vi "F5xxx Set Level.vi"(8 "error in (no error)":errorcluster, 9 "level [V/A]":dbl format="%^.3e", 10 "f [Hz]":dbl min=0.0 max=1200000.0 format="%^.3e", 11 "session in":T1) -> (0 "error out":errorcluster, 3 "session out":T1)   [LabVIEW 2020]
doc: "Set Fluke 5xxx voltage or current level."
uses:
  F5xxx_session.ctl
  F5xxx_output_mode.ctl
  Fluke 5XXX Series Multicalibrators.lvlib
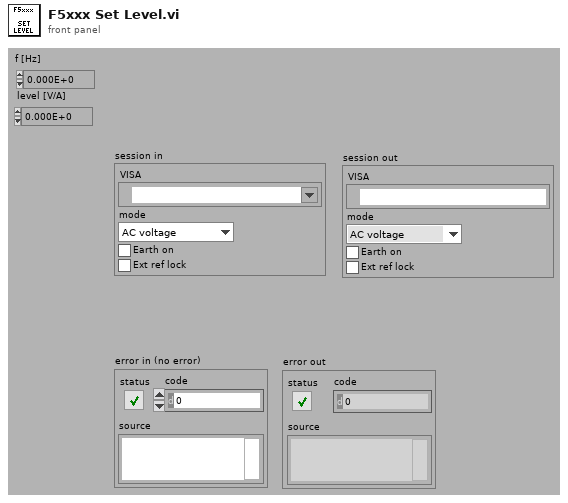
[diagram p1: front panel]
types:
  T1 = typedef "F5xxx_session.ctl" = cluster{"VISA":refnum<visa-resource-name>, "mode":T2, "Earth on":bool, "Ext ref lock":bool}
  T2 = typedef "F5xxx_output_mode.ctl" = enum16{"AC voltage", "AC current"}
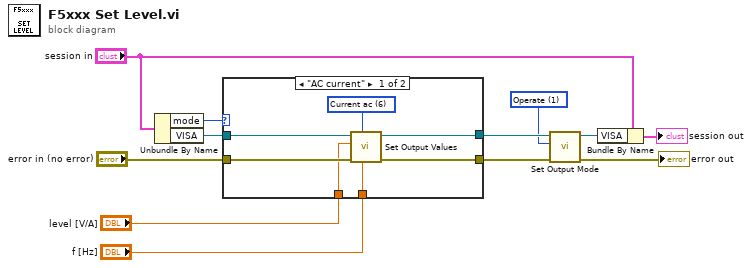
[diagram p0: block diagram]
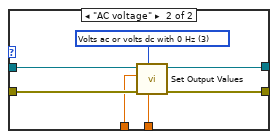
[diagram p2: hidden frame]
diagram:
  w1 = u32 1 items=["Standby", "Operate"] ("Output Mode (0: Standby)")
  n1 = Unbundle By Name("session in") -> ("mode"=w10:T2, "VISA"=w8:refnum<visa-resource-name>)
  n2 = case shown="\"AC current\"" w10 {
    tunnel: "error in (no error)" -> [w19 w26]
    tunnel: w8 -> [w18 w25]
    tunnel: "f [Hz]" -> [w17 w24]
    tunnel: "level [V/A]" -> [w15 w22]
    tunnel: [w14 w21] -> w5
    tunnel: [w13 w20] -> w4
    frame "AC current" {
      w16 = u32 6 items=["Amplitude", "Volts dc or update volts ac", "Volts ac dBm update", "Volts ac or volts dc with 0 Hz", "Volts ac in dBm", "Current dc or update current ac", "Current ac", "Update frequency", "Resistance", "Capacitance", "Temperature (Celsius)", "Temperature (Fahrenheit)", "Power dc or update power ac", "Power ac", "Dual volts dc or update dual ac", "Dual volts ac in volts", "Power ac in dBm update", "Power ac in dBm", "Dual volts ac in dBm update", "Dual volts ac in dBm"] ("Output Value(s) (0 - Amplitude)")
      n3 = call "Set Output Values.vi"("Fundamental Frequency (0.0 Hz)"=w17, "Output Value(s) (0 - Amplitude)"=w16, "error in (no error)"=w19, "Primary Value (0.0)"=w15, "VISA resource name"=w18) -> ("error out"=w14:errorcluster, "VISA resource name out"=w13:refnum<visa-resource-name>)  [unwired: 5 in]
    }
    frame "AC voltage" {
      w23 = u32 3 items=["Amplitude", "Volts dc or update volts ac", "Volts ac dBm update", "Volts ac or volts dc with 0 Hz", "Volts ac in dBm", "Current dc or update current ac", "Current ac", "Update frequency", "Resistance", "Capacitance", "Temperature (Celsius)", "Temperature (Fahrenheit)", "Power dc or update power ac", "Power ac", "Dual volts dc or update dual ac", "Dual volts ac in volts", "Power ac in dBm update", "Power ac in dBm", "Dual volts ac in dBm update", "Dual volts ac in dBm"] ("Output Value(s) (0 - Amplitude)")
      n4 = call "Set Output Values.vi"("Fundamental Frequency (0.0 Hz)"=w24, "Output Value(s) (0 - Amplitude)"=w23, "error in (no error)"=w26, "Primary Value (0.0)"=w22, "VISA resource name"=w25) -> ("error out"=w21:errorcluster, "VISA resource name out"=w20:refnum<visa-resource-name>)  [unwired: 5 in]
    }
  }
  n5 = call "Set Output Mode.vi"("error in (no error)"=w5, "Output Mode (0: Standby)"=w1, "VISA resource name"=w4) -> ("error out"=→"error out":errorcluster, "VISA resource name out"=w2:refnum<visa-resource-name>)  [unwired: 7 in]
  n6 = Bundle By Name(cluster="session in", "VISA"=w2) -> (→"session out":T1)
